vi "Check For Broken VIs.vi"(7 "before build?":bool, 8 "error in (no error)":errorcluster, 10 "Top-Level VIs":refnum<vi>[](array[refnum]), 11 "Class in":refnum<class "AB_SourceDistribution.lvclass">) -> (0 "error out":errorcluster, 3 "Class out":refnum<class "AB_SourceDistribution.lvclass">)   [LabVIEW 2020, in "AB_SourceDistribution.lvclass"]
uses:
  <vilib>/AppBuilder/AB_Classes/SourceDistribution/AB_SourceDistribution.lvclass
  e:/builds/penguin/labview/branches/2020/dev/dist/vi.lib/AppBuilder/AB_Classes/Build/AB_Build.lvclass
  <vilib>/AppBuilder/AB_Classes/Build/AB_Build.lvclass
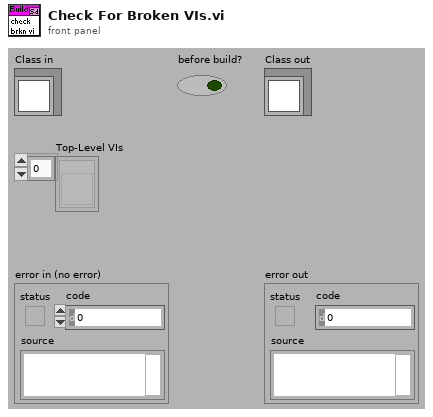
[diagram p1: front panel]
types:
  T1 = enum32{"Bad", "Idle", "Run top level", "Running"}
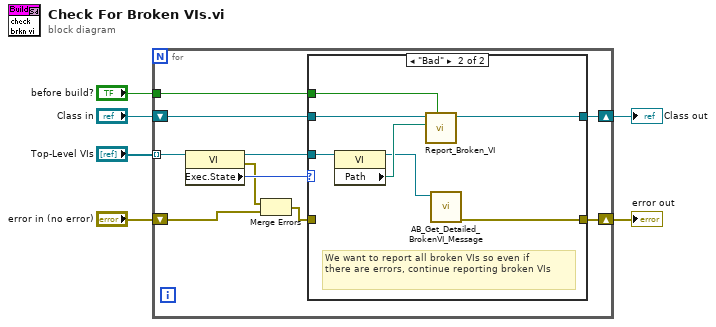
[diagram p0: block diagram]
diagram:
  n1 = for {
    shift-right: [w16] -> w3
    shift-left: "error in (no error)" -> [w8]
    shift-right: [w12] -> w4
    shift-left: "Class in" -> [w13]
    tunnel: "Top-Level VIs" -> [w11] mode=indexing
    tunnel: "before build?" -> [w7]
    n2 = property class="VI"(reference=w11) -> (reference out=w14:refnum<vi>, error out=w10:errorcluster, "Exec.State"=w15:T1)  [unwired: 1 in]
    n3 = Merge Errors(w10, w8) -> (w9:errorcluster)
    n4 = case shown="\"Bad\"" w15 {
      tunnel: w14 -> [_ w20]
      tunnel: [w18 w21] -> w16
      tunnel: w9 -> [w18 _]
      tunnel: w13 -> [w17 w24]
      tunnel: [w17 w23] -> w12
      tunnel: w7 -> [_ w22]
      frame Default {
      }
      frame "Bad" {
        # "We want to report all broken VIs so even if \nthere are errors, continue reporting broken VIs"
        n5 = property class="VI"(reference=w20) -> (reference out=w19:refnum<vi>, "Path"=w25:path)  [unwired: 1 in, 1 out]
        n6 = call <vilib>:"Report_Broken_VI.vi"("before build?"=w22, "vi path"=w25, "Build in"=w24) -> ("Build out"=w23:refnum<class "AB_SourceDistribution.lvclass">)  [unwired: 7 in, 1 out]
        n7 = call <vilib>:"AB_Get_Detailed_BrokenVI_Message.vi"("VI refnum"=w19) -> ("error out"=w21:errorcluster)  [unwired: 10 in]
      }
    }
  }
  "Class out" <- w4
  "error out" <- w3
